vi "Post-Build Action.vi"(5 "Files Generated by Build":path[](array[path]), 6 "Top Level/Always Included VIs":path[](array[path]), 7 "Destination Path":path, 8 "error in (no error)":errorcluster, 9 "Target Name":string, 10 "Build Specification Name":string, 11 "Project Path":path) -> (0 "error out":errorcluster)   [LabVIEW 2014, in "Oqus Custom Device.lvlib"]
uses:
  Oqus Custom Device.lvlib
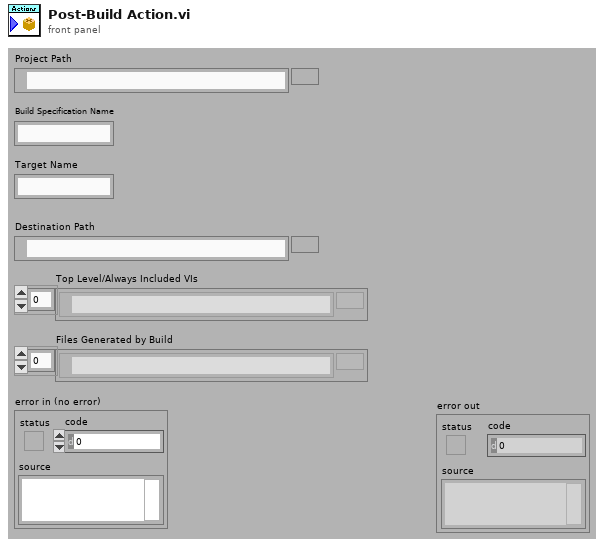
[diagram p1: front panel]
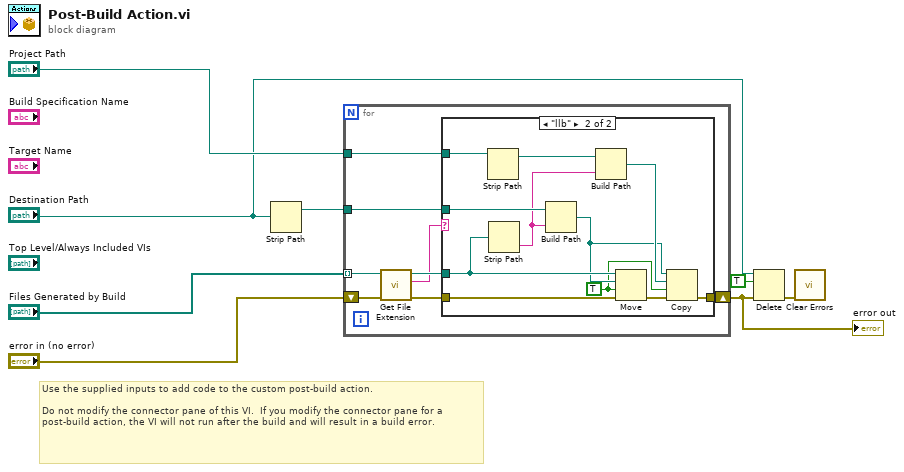
[diagram p0: block diagram]
diagram:
  # "Use the supplied inputs to add code to the custom post-build action.\n\nDo not modify the connector pane of this VI.  If you modify the connector pane for a post-build action, the VI will not run after the build and will result in a build error."
  n1 = Strip Path(path="Destination Path") -> (stripped path=w8:path)  [unwired: 1 out]
  n2 = for {
    tunnel: "Files Generated by Build" -> [w12] mode=indexing
    tunnel: w8 -> [w16]
    shift-right: [w15] -> w1
    shift-left: "error in (no error)" -> [w14]
    tunnel: "Project Path" -> [w9]
    n3 = call <vilib>:"Get File Extension.vi"("error in (no error)"=w14, "file"=w12) -> ("error out"=w13:errorcluster, "lowercase file extension"=w10:string, "dup file"=w11:path)  [unwired: 6 in, 1 out]
    n4 = case shown="\"llb\"" w10 {
      tunnel: w16 -> [_ w28]
      tunnel: [w17 w18] -> w15
      tunnel: w13 -> [w17 w26]
      tunnel: w11 -> [_ w27]
      tunnel: w9 -> [_ w24]
      frame Default {
      }
      frame "llb" {
        w20 = TRUE ("overwrite (F)")
        n5 = Strip Path(path=w24) -> (stripped path=w25:path)  [unwired: 1 out]
        n6 = Strip Path(path=w27) -> (name=w23:string)  [unwired: 1 out]
        n7 = Build Path(base path=w28, name or relative path=w23) -> (appended path=w21:path)
        n8 = Build Path(base path=w25, name or relative path=w23) -> (appended path=w22:path)
        n9 = Move(source path=w27, error in=w26, 9:w20, 10:w21) -> (error out=w19:errorcluster)  [unwired: 1 in, 2 out]
        n10 = Copy(8:w19, 9:w20, 10:w22, 11:w21) -> (0:w18:errorcluster)  [unwired: 1 in, 2 out]
      }
    }
  }
  "error out" <- w1
  n11 = Delete(path (use dialog)="Destination Path", entire hierarchy (F)=TRUE, error in=w1) -> (error out=w7:errorcluster)  [unwired: 2 in, 2 out]
  n12 = call <vilib>:"Clear Errors.vi"("error in (no error)"=w7) -> ()  [unwired: 5 in, 2 out]
